vi "Close.vi"(8 "error in":errorcluster, 11 "Tacmina Settings in":T1) -> (0 "error out":errorcluster, 3 "Tacmina Settings out":T1)   [LabVIEW 2018, in "Tacmina QI.lvlib"]
uses:
  Tacmina QI.lvlib
  Tacmina QI DAQ Setting.ctl
  <vilib>/DAQmx/write.llb/DAQmx Write (Digital Bool 1Line 1Point).vi
  <vilib>/DAQmx/miscellaneous.llb/DAQmx Fill In Error Info.vi
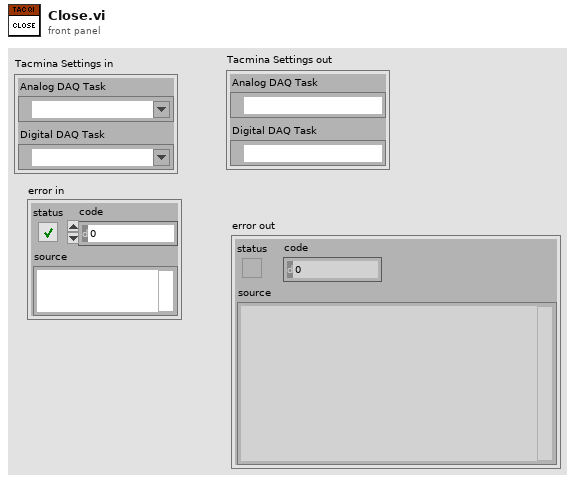
[diagram p1: front panel]
types:
  T1 = typedef "Tacmina QI.lvlib/Tacmina QI DAQ Setting.ctl" = cluster{"Analog DAQ Task":refnum<k21>, "Digital DAQ Task":refnum<k21>}
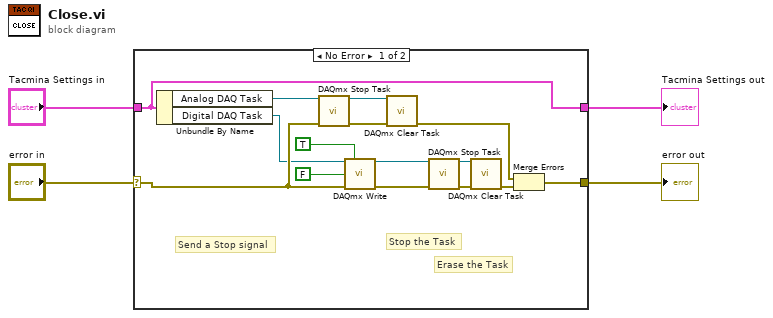
[diagram p0: block diagram]
diagram:
  n1 = case shown="No Error" "error in" {
    selector: "error in" -> [w8 w21]
    tunnel: [w12 w21] -> w3
    tunnel: "Tacmina Settings in" -> [w5 w20]
    tunnel: [w5 w20] -> w1
    frame No Error {
      # "Erase the Task"
      # "Stop the Task"
      # "Send a Stop signal"
      n2 = Unbundle By Name(w5) -> ("Analog DAQ Task"=w15:refnum<k21>, "Digital DAQ Task"=w7:refnum<k21>)
      n3 = call <vilib>:"DAQmx Stop Task.vi"("task/channels in"=w15, "error in"=w8) -> ("task out"=w16:refnum<k21>, "error out"=w17:errorcluster)  [unwired: 12 in]
      n4 = call-poly <vilib>:"DAQmx Write.vi"("task/channels in"=w7, "auto start"=TRUE, "data"=FALSE, "error in"=w8) -> ("task out"=w6:refnum<k21>, "error out"=w9:errorcluster)  [unwired: 9 in, 1 out]
      n5 = call <vilib>:"DAQmx Clear Task.vi"("task in"=w16, "error in"=w17) -> ("error out"=w13:errorcluster)  [unwired: 13 in]
      n6 = call <vilib>:"DAQmx Stop Task.vi"("task/channels in"=w6, "error in"=w9) -> ("task out"=w19:refnum<k21>, "error out"=w18:errorcluster)  [unwired: 12 in]
      n7 = call <vilib>:"DAQmx Clear Task.vi"("task in"=w19, "error in"=w18) -> ("error out"=w14:errorcluster)  [unwired: 13 in]
      n8 = Merge Errors(w13, w14) -> (w12:errorcluster)
    }
    frame Error {
    }
  }
  "error out" <- w3
  "Tacmina Settings out" <- w1
